vi "python_pattern.vi"(3 "Python error in":errorcluster, 4 "Pattern Definition":T2={"Spot pitch (pixels)"=23.1, "Tilt Angle (deg)"=0.0, "Horizontal Offset (pixels)"=91.9, "Vertical Offset (pixels)"=14.1, "# Horizontal Spots"=8, "# Vertical Spots"=1, "Spot size (pixels)"=23.1, "Darken center spot"=FALSE, "Exact Phase Formula"=TRUE, "phase wrapping"=FALSE, "Set Focus (mm)"=32.0, "Add phase"=4.0, "phase_factor"=65.0, "Steering LW"=2.0, "Steering vmax"=0.0, "phase_overshoot"=TRUE, "Focal shift param"=0.0, "x0 focal shift"=0.0, "y0 focal shift"=0.0, "hv_steering"=TRUE, "fixed"=TRUE, "Pad"=0.0, "dark_all"=FALSE, "nospot"=FALSE, "Laser wavelength"=6.28e-07} {"Laser wavelength" min=0.0 max=500.0 format="%^#.3e"; "Pad" min=0.0 max=500.0 step=1.0 format="%#.0g"; "y0 focal shift" min=0.0 max=500.0 format="%#.3g"; "x0 focal shift" min=0.0 max=500.0 format="%#.3g"; "Focal shift param" min=0.0 max=500.0 format="%#.3g"; "Steering vmax" min=0.0 max=500.0 format="%#.3g"; "Steering LW" min=0.0 max=500.0 format="%#.3g"; "phase_factor" min=0.0 max=500.0 format="%#.3f"; "Add phase" min=0.0 max=500.0 format="%#.3f"; "Set Focus (mm)" min=0.0 max=500.0 format="%#.3g"; "Spot size (pixels)" min=1.0 format="%.2g"; "# Vertical Spots" min=1 step=1; "# Horizontal Spots" min=1 step=1; "Vertical Offset (pixels)" format="%.2f"; "Horizontal Offset (pixels)" format="%.2f"; "Tilt Angle (deg)" min=-90.0 max=90.0 format="%.2g"; "Spot pitch (pixels)" min=1.0 format="%.2g"}, 5 "Python Session in":T1=refnum) -> (0 "Python error out":errorcluster={"status"=TRUE, "code"=1050, "source"="PYTHON Execute Script__ogtk.vi->mulitspot_pattern_static3_session.vi->test_mulitspot_pattern_static3_session.vi:<type 'exceptions.NameError'>, global name 'np' is not defined"}, 1 "Float Matrix":dbl[][](array[numeric]), 2 "Python Session out":T1)   [LabVIEW 2011]
uses:
  Periodic Spot Pattern Parameters.ctl
  Periodic Spot Pattern Parameters2.ctl
  <userlib>/_OpenG.lib/labpython/labpython.llb/PYTHON Session Refnum__ogtk.ctl
  <userlib>/_OpenG.lib/labpython/labpython.llb/PYTHON Set Float Vector__ogtk.vi
  <userlib>/_OpenG.lib/labpython/labpython.llb/PYTHON Set Float Data__ogtk.vi
  <userlib>/_OpenG.lib/labpython/labpython.llb/PYTHON Set Integer Data__ogtk.vi
  <userlib>/_OpenG.lib/labpython/labpython.llb/PYTHON Set Boolean Data__ogtk.vi
  <userlib>/_OpenG.lib/labpython/labpython.llb/PYTHON Get Float Matrix__ogtk.vi
  <userlib>/_OpenG.lib/labpython/labpython.llb/PYTHON Get String Data__ogtk.vi
panel:
  in  "Debug":bool
  out "Loaded script":string
  out "File error out":errorcluster
  in  "Script path":path=path "C:/Data/Antonio/software/LCOS/LCOS_CompleteLV/python/pattern_labview_session_script.py"
  in  "center_spot (to be darkened)":u16=4
  out "A string (just debug)":string
  out "Xm":dbl[](array[numeric])=[21.72, 44.87, 68.2, 91.45, 114.72, 137.87, 160.97, 184.04]
  in  "Xm String (csv)":string="21.72,  44.87,  68.20,  91.45, 114.72, 137.87, 160.97, 184.04"
  out "Ym":dbl[](array[numeric])=[13.84, 23.78, 13.79, 13.83, 13.75, 13.79, 13.74, 13.68]
  in  "Ym String (csv)":string="13.84,  23.78,  13.79,  13.83,  13.75,  13.79,  13.74,  13.68"
  out "Intensity Graph":dbl[][](graph)
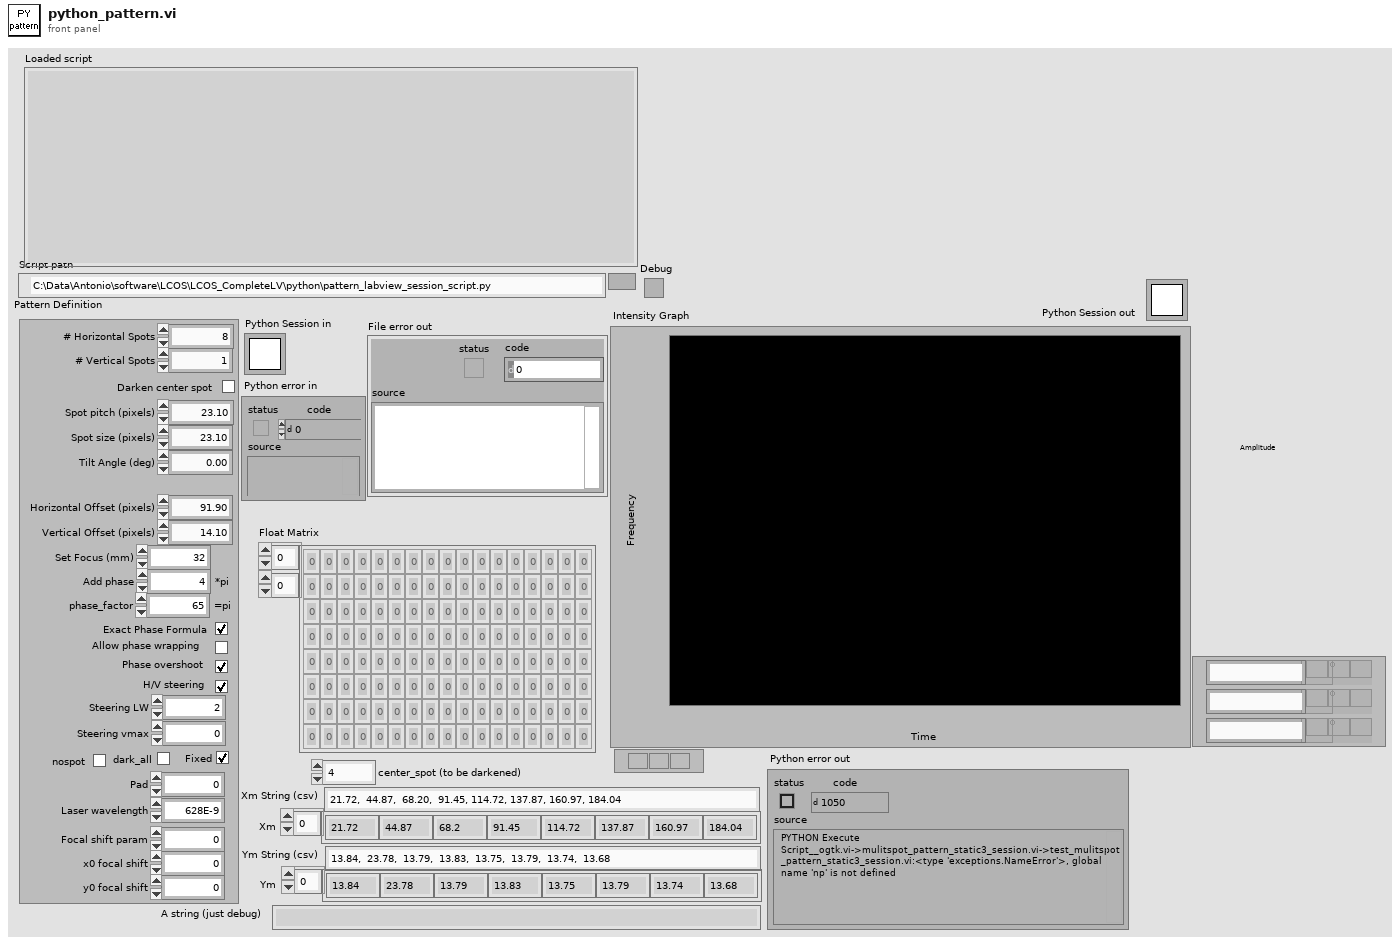
[diagram p1: front panel]
types:
  T1 = typedef "PYTHON Session Refnum__ogtk.ctl" = refnum<k1>
  T2 = typedef "Periodic Spot Pattern Parameters.ctl" = cluster{"Spot pitch (pixels)":dbl, "Tilt Angle (deg)":dbl, "Horizontal Offset (pixels)":dbl, "Vertical Offset (pixels)":dbl, "# Horizontal Spots":u32, "# Vertical Spots":u32, "Spot size (pixels)":dbl, "Darken center spot":bool, "Exact Phase Formula":bool, "phase wrapping":bool, "Set Focus (mm)":T3, "Add phase":dbl, "phase_factor":dbl, "Steering LW":T3, "Steering vmax":T3, "phase_overshoot":bool, "Focal shift param":T3, "x0 focal shift":T3, "y0 focal shift":T3, "hv_steering":bool, "fixed":bool, "Pad":T3, "dark_all":bool, "nospot":bool, "Laser wavelength":dbl}
  T3 = typedef "Periodic Spot Pattern Parameters2.ctl" = dbl
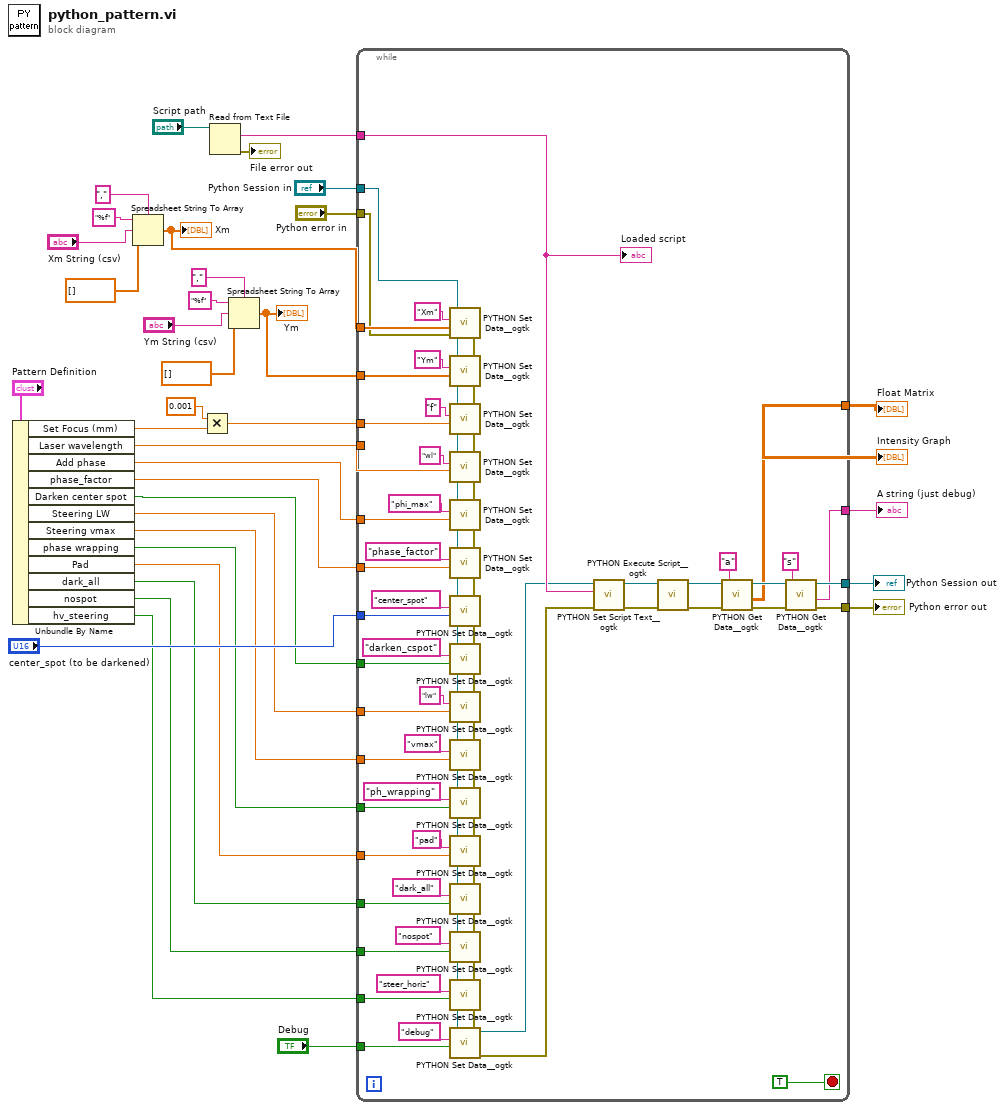
[diagram p0: block diagram]
diagram:
  n1 = Unbundle By Name("Pattern Definition") -> ("Set Focus (mm)"=w27:T3, "Laser wavelength"=w22:dbl, "Add phase"=w21:dbl, "phase_factor"=w20:dbl, "Darken center spot"=w18:bool, "Steering LW"=w17:T3, "Steering vmax"=w16:T3, "phase wrapping"=w15:bool, "Pad"=w14:T3, "dark_all"=w13:bool, "nospot"=w12:bool, "hv_steering"=w2:bool)
  n2 = Spreadsheet String To Array(delimiter (Tab)=",", format string="%f", spreadsheet string="Xm String (csv)", array type (2D Dbl)=dbl[] []) -> (array=w25:dbl[])
  "Xm" <- w25
  n3 = Multiply(x=T3 0.001, y=w27) -> (x*y=w23:T3)
  n4 = Read from Text File(file (use dialog)="Script path") -> (text=w10:string, error out=→"File error out":errorcluster)  [unwired: 3 in, 2 out]
  n5 = Spreadsheet String To Array(delimiter (Tab)=",", format string="%f", spreadsheet string="Ym String (csv)", array type (2D Dbl)=dbl[] []) -> (array=w24:dbl[])
  "Ym" <- w24
  n6 = while {
    tunnel: w25 -> [w76]
    tunnel: w24 -> [w75]
    tunnel: w23 -> [w74]
    tunnel: w22 -> [w73]
    tunnel: w21 -> [w72]
    tunnel: w20 -> [w71]
    tunnel: "center_spot (to be darkened)" -> [w70]
    tunnel: w18 -> [w69]
    tunnel: w17 -> [w68]
    tunnel: w16 -> [w67]
    tunnel: w15 -> [w66]
    tunnel: w14 -> [w65]
    tunnel: w13 -> [w64]
    tunnel: w12 -> [w63]
    tunnel: w10 -> [w56]
    tunnel: [w53] -> w8
    tunnel: [w52] -> w7
    tunnel: [w51] -> w6
    tunnel: [w50] -> w5
    tunnel: "Python Session in" -> [w49]
    tunnel: "Python error in" -> [w48]
    tunnel: w2 -> [w43]
    tunnel: "Debug" -> [w37]
    stop <- TRUE ("stop") stop-if-true
    n7 = call-poly <userlib>:"PYTHON Set Data__ogtk.vi"("error in (no error)"=w48, "value"=w76, "variable name"="Xm", "Python Session in"=w49) -> ("error out"=w105:errorcluster, "Python Session out"=w116:T1)  [unwired: 2 in]
    n8 = call-poly <userlib>:"PYTHON Set Data__ogtk.vi"("error in (no error)"=w105, "value"=w75, "variable name"="Ym", "Python Session in"=w116) -> ("error out"=w104:errorcluster, "Python Session out"=w115:T1)  [unwired: 2 in]
    n9 = call-poly <userlib>:"PYTHON Set Data__ogtk.vi"("error in (no error)"=w104, "value"=w74, "variable name"="f", "Python Session in"=w115) -> ("error out"=w103:errorcluster, "Python Session out"=w114:T1)  [unwired: 2 in]
    n10 = call-poly <userlib>:"PYTHON Set Data__ogtk.vi"("error in (no error)"=w103, "value"=w73, "variable name"="wl", "Python Session in"=w114) -> ("error out"=w102:errorcluster, "Python Session out"=w113:T1)  [unwired: 2 in]
    n11 = call-poly <userlib>:"PYTHON Set Data__ogtk.vi"("error in (no error)"=w102, "value"=w72, "variable name"="phi_max", "Python Session in"=w113) -> ("error out"=w101:errorcluster, "Python Session out"=w112:T1)  [unwired: 2 in]
    n12 = call-poly <userlib>:"PYTHON Set Data__ogtk.vi"("error in (no error)"=w101, "value"=w71, "variable name"="phase_factor", "Python Session in"=w112) -> ("error out"=w100:errorcluster, "Python Session out"=w111:T1)  [unwired: 2 in]
    n13 = call-poly <userlib>:"PYTHON Set Data__ogtk.vi"("error in (no error)"=w100, "value"=w70, "variable name"="center_spot", "Python Session in"=w111) -> ("error out"=w99:errorcluster, "Python Session out"=w110:T1)  [unwired: 2 in]
    n14 = call-poly <userlib>:"PYTHON Set Data__ogtk.vi"("error in (no error)"=w99, "value"=w69, "variable name"="darken_cspot", "Python Session in"=w110) -> ("error out"=w98:errorcluster, "Python Session out"=w109:T1)  [unwired: 2 in]
    n15 = call-poly <userlib>:"PYTHON Set Data__ogtk.vi"("error in (no error)"=w98, "value"=w68, "variable name"="lw", "Python Session in"=w109) -> ("error out"=w97:errorcluster, "Python Session out"=w108:T1)  [unwired: 2 in]
    n16 = call-poly <userlib>:"PYTHON Set Data__ogtk.vi"("error in (no error)"=w97, "value"=w67, "variable name"="vmax", "Python Session in"=w108) -> ("error out"=w96:errorcluster, "Python Session out"=w107:T1)  [unwired: 2 in]
    n17 = call-poly <userlib>:"PYTHON Set Data__ogtk.vi"("error in (no error)"=w96, "value"=w66, "variable name"="ph_wrapping", "Python Session in"=w107) -> ("error out"=w81:errorcluster, "Python Session out"=w106:T1)  [unwired: 2 in]
    n18 = call-poly <userlib>:"PYTHON Set Data__ogtk.vi"("error in (no error)"=w81, "value"=w65, "variable name"="pad", "Python Session in"=w106) -> ("error out"=w80:errorcluster, "Python Session out"=w78:T1)  [unwired: 2 in]
    n19 = call-poly <userlib>:"PYTHON Set Data__ogtk.vi"("error in (no error)"=w80, "value"=w64, "variable name"="dark_all", "Python Session in"=w78) -> ("error out"=w79:errorcluster, "Python Session out"=w77:T1)  [unwired: 2 in]
    n20 = call-poly <userlib>:"PYTHON Set Data__ogtk.vi"("error in (no error)"=w79, "value"=w63, "variable name"="nospot", "Python Session in"=w77) -> ("error out"=w44:errorcluster, "Python Session out"=w45:T1)  [unwired: 2 in]
    n21 = call-poly <userlib>:"PYTHON Set Data__ogtk.vi"("error in (no error)"=w44, "value"=w43, "variable name"="steer_horiz", "Python Session in"=w45) -> ("error out"=w41:errorcluster, "Python Session out"=w42:T1)  [unwired: 2 in]
    n22 = call-poly <userlib>:"PYTHON Set Data__ogtk.vi"("error in (no error)"=w41, "value"=w37, "variable name"="debug", "Python Session in"=w42) -> ("error out"=w39:errorcluster, "Python Session out"=w40:T1)  [unwired: 2 in]
    n23 = call <userlib>:"PYTHON Set Script Text__ogtk.vi"("error in (no error)"=w39, "script text"=w56, "Python Session in"=w40) -> ("error out"=w59:errorcluster, "Python Session out"=w62:T1)  [unwired: 3 in]
    n24 = call <userlib>:"PYTHON Execute Script__ogtk.vi"("error in (no error)"=w59, "Python Session in"=w62) -> ("error out"=w58:errorcluster, "Python Session out"=w61:T1)  [unwired: 4 in]
    n25 = call-poly <userlib>:"PYTHON Get Data__ogtk.vi"("error in (no error)"=w58, "variable name"="a", "Python Session in"=w61) -> ("error out"=w57:errorcluster, "value"=w50:dbl[][], "Python Session out"=w60:T1)  [unwired: 2 in]
    n26 = call-poly <userlib>:"PYTHON Get Data__ogtk.vi"("error in (no error)"=w57, "variable name"="s", "Python Session in"=w60) -> ("error out"=w52:errorcluster, "value"=w51:string, "Python Session out"=w53:T1)  [unwired: 2 in]
    "Loaded script" <- w56
  }
  "Float Matrix" <- w5
  "Intensity Graph" <- w5
  "A string (just debug)" <- w6
  "Python Session out" <- w8
  "Python error out" <- w7
